vi "ConstantForce.vi"() -> ()   [LabVIEW 2011]
doc: "This example is a template that gives the structure of a single-loop PID controller. This VI uses the PID Filter VI to reduce measurement noise. This VI also uses the PID Autotuning VI to tune the controller based on the closed-loop response. This VI also uses the Timed Loop to ensure deterministic execution.\n\nReplace the Dummy Input and Dummy Output VIs with code that communicates with a real-time target."
uses:
  <vilib>/addons/Digital Filter Design/_Objects.llb/DFD Filter Obj.ctl
  <vilib>/addons/Digital Filter Design/_Objects.llb/DFD Filter Coef.ctl
  <vilib>/addons/Digital Filter Design/_Objects.llb/DFD Filter Structure Type Selector.ctl
  <vilib>/addons/Digital Filter Design/_Objects.llb/dfd_Internal Quantization Settings.ctl
  <vilib>/addons/Digital Filter Design/_Objects.llb/dfd_Internal Quantization Srcs.ctl
  <vilib>/addons/Digital Filter Design/_Objects.llb/DFD Coef Norm Type.ctl
  <vilib>/Platform/TimedLoop/XDataNode/timing_clust.ctl
  <vilib>/Platform/TimedLoop/XDataNode/nitl_modes.ctl
  <vilib>/Platform/TimedLoop/XDataNode/wakeup.ctl
  <vilib>/DAQmx/write.llb/DAQmx Write (Counter Frequency 1Chan 1Samp).vi
  <vilib>/DAQmx/write.llb/DAQmx Write (Digital 1D Bool NChan 1Samp 1Line).vi
  <vilib>/DAQmx/read.llb/DAQmx Read (Counter DBL 1Chan 1Samp).vi
  <vilib>/DAQmx/read.llb/DAQmx Read (Analog 1D DBL NChan 1Samp).vi
  <vilib>/addons/control/pid/pid.llb/PID Advanced (DBL Array).vi
  <vilib>/addons/control/pid/pid.llb/PID Derivative Action Buffered (DBL Array).vi
  <vilib>/addons/control/pid/pid.llb/PID Get Advanced Error (DBL Array).vi
  <vilib>/addons/control/pid/pid.llb/PID Integral Action Buffered (DBL Array).vi
  <vilib>/addons/control/pid/pid.llb/PID Resize 1D Array.vi
  <vilib>/addons/control/pid/pid.llb/PID Get Advanced Error (DBL).vi
  <vilib>/DAQmx/create/channels.llb/DAQmx Create Channel (CO-Pulse Generation-Frequency).vi
  <vilib>/DAQmx/configure/timing.llb/DAQmx Timing (Implicit).vi
  <vilib>/DAQmx/miscellaneous.llb/DAQmx Fill In Error Info.vi
  <vilib>/addons/Digital Filter Design/Process.llb/DFD Filtering (PtByPt NChan).vi
  <vilib>/addons/control/pid/pid.llb/PID Parameter Manager (DBL Array).vi
  <vilib>/measure/maspectr.llb/FFT Spectrum (Mag-Phase) for 1 Chan.vi
  <vilib>/Platform/TimedLoop/XDataNode/XDataNode.xnode
  <vilib>/Platform/TimedLoop/XDataNode/XDNodeRunTimeDep.lvlib
  <vilib>/addons/Digital Filter Design/NI_DigFilterLicensed.lvlib
  <vilib>/measure/NI_MAPro.lvlib
  <vilib>/Analysis/NI_AAL_SigProc.lvlib
  <vilib>/addons/control/pid/NI_PID_pid.lvlib
panel:
  in  "linearity":dbl=1.0 format="%.2f"
  out "PIDGainsOut":T1(array[cluster])=[{"proportional gain (Kc)"=0.30000000000000004, "integral time (Ti, min)"=0.0, "derivative time (Td, min)"=0.0}, {"proportional gain (Kc)"=0.30000000000000004, "integral time (Ti, min)"=0.0, "derivative time (Td, min)"=0.0}, {"proportional gain (Kc)"=0.30000000000000004, "integral time (Ti, min)"=0.0, "derivative time (Td, min)"=0.0}]
  in  "PIDGains":T2={"proportional high (Kc)"=0.5, "integral high (Ti, min)"=0.0, "derivative high (Td, min)"=0.0, "derivative low (Td, min)"=0.0, "integral low (Ti, min)"=0.0, "proportional low (Kc)"=0.1}
  in  "PWMFreq(Hz)":dbl=20000.0 format="%#.6f"
  out "Spectrum":cluster{"f0":dbl, "df":dbl, "magnitude":dbl[]}(graph)={"f0"=0.0, "df"=0.5, "magnitude"=[0.09620328441748356, 0.06810409897269343, 0.0003594915796713484, 0.00021014860402491955, 0.00018846954399764898, 0.000336144679529325, 0.0003012130801723677, 0.00019445462332171186, 0.00033289517846645525, 0.000562837200884615, 0.0006867747058623169, 0.0005811212987675227, 0.00042648431087789106, 0.00036723054948810537, 0.0005888304364960171, 0.0003765129395675796, 0.0002678403496865518, 0.00026380175267942224, 0.000361787601543214, 0.0001537222322813939, 0.0004248104230093206, 0.000271774297036959, 0.00019403766325024087, 7.837182938118593e-05, 0.00024086646260639623, 0.00021325629753186142, 0.00035497074211725515, 0.0005320390408672116, 0.0005154588307424057, 0.000495977514915726, 0.0001925926892680212, 0.00019634614136678798, 0.00046755672378875993, 0.00021183899474091903, 0.000356482164933941, 0.0005724397171551199, 0.0006112453042765386, 0.00014832611393915694, 0.0005354449091516573, 0.0002972453160266781, 0.00017597805789222284, 0.00032530655361426877, 0.00014118024452655864, 0.00036010109356104285, 0.000578316221003946, 0.0007461816021521776, 0.0008385140163832047, 0.0004886726202003539, 0.0003150315464376134, 0.000525543904177902, 0.00041318124423732366, 0.0003192525289590377, 0.00044682022013315406, 0.00023378315775143073, 0.0004028294060579752, 0.00016764084886402385, 0.0002658689552949207, 0.00011811227072949446, 0.0005108675726238193, 0.000528660037898421, 0.0004661368639780102, 0.0001969172989955398, 0.0002997817435090788, 0.0005232481265916394, 0.00029153354829127535, 0.00034458564082988065, 0.0003625549267826836, 0.00030485399320604465, 2.100427401405029e-05, 0.00033163055233150494, 0.0002575243373899191, 0.00031024447712355024, 0.0007095809580562265, 0.0005526875168590069, 0.00018836331735285066, 0.0003619452686631739, 0.0004012983928592705, 0.0003666381061545948, 0.000163582673291403, 0.00012291988292315167, 0.00015891526892010527, 0.00030324875662186086, 0.0001862711270856599, 0.0002485152285499018, 0.0010135478143531338, 0.0008078916475509933, 0.00019359871503329563, 0.000242729443732801, 0.0003349348406560765, 9.595394744410574e-05, 0.00025533462003401097, 0.0001751733067829238, 0.00021051280903753254, 0.0005121321454423101, 0.00027114121521858316, 0.00015587679564032464, 5.8841200038904936e-05, 0.00020608135420260734, 0.00011735729480533824, 0.00010462900746872218, 0.0001985190237984826, 0.00022073477853828147, 0.0003930499011930387, 0.00015089927914282338, 0.00017461102815684548, 0.00036546505890260473, 0.0004575643420051038, 6.526037412657404e-05, 0.00023842870451437197, 0.00022795175255096854, 0.00018803736048158008, 0.00043762334105444596, 0.00037204602762833686, 0.0003858127901442611, 0.00019537399379967473, 0.00030700211982774474, 0.00023405998375632787, 0.0003412354867453395, 0.00030349101678903823, 0.0005609930012192304, 0.0005962425745295062, 0.0022891501106861896, 0.001532704893945848, 0.00038033835660364, 0.0006200757374118415, 0.0004930594092931169, 0.00024339834621575263, 0.0003658239842420277, 0.0005250237628612773, 0.0003061662633654362, 0.0004469940702075021, 0.00045614841528136314, 0.00026832273527844684, 0.0005091044695006741, 0.0003169947020805991, 0.00023486424468684847, 8.763839647824092e-05, 0.00012753416525012625, 0.0003161495448484612, 2.4514922051848186e-05, 0.0002764823360063886, 0.0001578650633790925, 0.00010584168072209294, 0.00014471171973597772, 0.00034066054923323106, 0.00013362866729409327, 0.00033852904863394633, 0.0003590766483400952, 0.00014033182697085645, 0.00011189728703164615, 0.00037718943519435576, 0.0003853277661842273, 0.0001247091613316533, 0.00015688449877991313, 0.0003789219713444136, 0.00018460493488254377, 0.0003119702921186279, 3.0397927282497637e-05, 0.0003359855665221087, 0.0004626969711366938, 0.0003920309415639225, 0.00013392270975849446, 8.86969666433672e-05, 0.00028416480332106846, 0.0004775515986091747, 0.00017753284475210284, 0.00024506374036664647, 0.00046639045447426954, 0.00046301499237699274, 9.541922668358468e-05, 0.0001347948324566838, 2.8572305924906603e-05, 0.00021058685814798146, 0.0003797764082673831, 0.00035629394402777965, 0.00032325251665472844, 0.00040608713555629743, 0.00026898733488955054, 0.0003224959059278195, 0.0004177458017480001, 0.0003681014963565972, 0.00021977425088954856, 0.00035957776746553847, 0.0003226402567141675, 0.00016441447267492444, 0.0002355870386269575, 0.0002162722984969486, 0.0001896749433490035, 4.427063644161406e-05, 0.0002739512902890422, 0.00057854822568849, 0.00033369187305485866, 0.000289470863002901, 8.046137507455306e-05, 0.00023404201343144298, 0.00019294437276071608, 6.054397015157805e-05, 0.00019065185856366197, 0.00027288045779204795, 0.00026849048114022014, 0.00025544691639125465, 0.00013667814777984988, 0.00031897709809037964, 0.0003167770003048542, 0.00018790987805623638, 0.00014065616466841214, 0.00027750941214549823, 0.00034764390165337514, 0.00016498491417466518, 0.00026200335705082545, 0.0002430179402840247, 0.00012993406172108322, 0.00011384517778497205, 0.00020210395661492624, 0.0001926177237363148, 0.0001566807843681054, 8.786807745152152e-05, 0.00011506274315827096, 0.00018052211173992514, 0.0003506426925901174, 0.0001150344595900169, 0.0002006531517296627, 0.00012199567861928173, 6.968881651603949e-05, 0.000146895434695057, 0.00010177868227619922, 7.146367819549118e-05, 0.00012302008869253934, 0.00015391572161203, 0.0003878908024648666, 0.00016205775672610318, 0.0003730406559238256, 0.0004949639629069069, 0.0002414474567828382, 6.715996397035274e-06, 0.0001982056525915547, 0.00017415448516628528, 0.00012697343205469538, 7.0467005193071e-05, 8.522897645077587e-05, 0.00011608238840935515, 0.00021737273984480314, 0.0002143539233942704, 0.0001547982432409731, 0.00013387049192060244, 0.00024362621289604044, 0.00025346685262303667, 0.00011828114208063182, 0.0001410973697475952, 0.00016484708553944803, 9.362003895362505e-05, 3.742238618907275e-05, 8.816624296788719e-05, 8.660419917454452e-05, 8.454844225543479e-05, 0.00014563770331394723, 0.00016165886336021103, 0.00029643091094315444, 0.00022617051620957054, 7.425864446578824e-05, 0.00012984973460739143, 0.00029941459060023215, 0.00019887115018064593, 0.0001550592860894656, 0.00010701912873426859, 5.644325495758224e-05, 0.00012987724039262955, 0.0001623444017767889, 0.0001245355197327217, 0.00014574362683201258, 2.5439415031698453e-05, 8.203135152081712e-05, 0.00011453414541864422, 1.5990912903028797e-05, 9.48759521834382e-05, 8.071394034967105e-05, 0.00017365760224407863, 0.00017999404550366962, 9.887670279700942e-05, 5.502379636777061e-05, 8.329224876693273e-05, 0.00011744377274604075, 0.00012808337474860536, 0.00017429621949908563, 6.559673716533871e-05, 8.517439602839222e-05, 5.581680993555922e-05, 0.0001248433166413104, 0.00011297876140050008, 0.00010607476864400097, 7.557647775344107e-05, 9.027165709926598e-05, 9.26301339988804e-05, 7.111166199659558e-05, 4.503125015873237e-05, 7.134205040841814e-05, 0.00017176642240616653, 0.00015805834772730266, 6.354909821912828e-05, 4.710721765108564e-05, 5.961174275940043e-05, 2.3994340360453395e-05, 2.9612149535282676e-05, 8.068837779654663e-05, 8.337468168258811e-05, 5.9948988957651735e-05, 1.2901070157195641e-05, 9.928627098209403e-05, 9.911589258071182e-05, 9.27104415452593e-05, 5.297783951889115e-05, 8.866164597341511e-05, 6.873540575424902e-05, 2.9752777982596516e-05, 0.00017445943670187227, 0.00024159254243468698, 0.00011658923271226115, 0.00012737326503517066, 0.0001389373667419545, 0.00010623090442469181, 7.523416408699585e-05, 7.220312378677459e-05, 3.864949977027068e-05, 4.515642057022097e-05, 5.204067025147724e-05, 9.064350175867587e-05, 5.107043973201085e-05, 0.0001245826862645853, 0.00010515742874481237, 4.752206290018221e-05, 0.00010955241723395005, 7.407898359610076e-05, 2.1708007746722337e-05, 2.019715590464164e-05, 2.1987406689666923e-05, 5.450113354923983e-05, 7.161957983578496e-05, 6.641173438069711e-05, 6.87976800359608e-05, 5.240743045604911e-05, 3.664493515963725e-05, 7.418481441817933e-05, 9.749743503975909e-05, 9.073727003872781e-05, 2.1989849094629526e-05, 5.746344157877747e-05, 1.8546935661777757e-05, 2.722942258343563e-05, 3.0658397698000485e-05, 9.776292178957533e-06, 1.2335863321959672e-05, 3.2727818473110664e-05, 1.3584172902497782e-05, 1.3556247846696258e-05, 1.2761952374912845e-05, 5.991948995900634e-05, 3.816873057478155e-05, 6.78400724612916e-05, 8.797430347711267e-05, 5.2462210266196544e-05, 1.058840890246386e-05, 2.5716730457104114e-05, 1.2751793024547623e-05, 1.6181032458945755e-05, 2.5965989392743585e-05, 4.399652423913049e-05, 5.88406679814353e-05, 3.9070027684511886e-05, 1.6725512968109914e-05, 1.0581280299026412e-05, 2.744399368794747e-05, 3.794992163132296e-05, 2.366887226580642e-05, 2.7508074750656194e-05, 3.317018088757152e-05, 1.866435406036027e-05, 1.1448271641135718e-05, 1.0825975855801427e-05, 1.9921166088270942e-05, 2.513310121648055e-05, 1.4239372227448338e-05, 1.9887056193184144e-05, 3.146587181328742e-06, 4.3519333042847355e-06, 1.633265643308589e-05, 1.3654781858151129e-05, 3.6984701177022112e-06, 4.393726542097977e-05, 4.816543678632307e-05, 2.734925118918193e-05, 2.1002282860069026e-05, 1.66693272371177e-05, 2.070731099804239e-05, 3.2537835380993076e-05, 2.419553306105436e-05, 4.797854579184654e-06, 2.2696380463346525e-05, 2.783896678820508e-05, 1.370374056458416e-05, 1.2943130388085828e-05, 1.1433275758105753e-05, 1.179814825411713e-05, 1.563252142645715e-05, 1.928199143307197e-05, 1.8918668232749954e-05, 1.1217316209080702e-05, 1.5511054495680417e-05, 6.777718332613398e-06, 1.8789937755635533e-05, 1.7817142540518592e-05, 1.2246089319170154e-05, 1.6629467750457185e-05, 2.051993540859729e-05, 2.098327932203105e-05, 6.057051820967863e-06, 6.714391983681018e-06, 6.356643139768899e-06, 8.45582646188679e-06, 5.622569738697892e-06, 1.101240684909168e-05, 1.4877549032696077e-05, 1.1375986593766988e-05, 2.1919217303393563e-05, 9.085871491365278e-06, 7.113283544734878e-06, 8.90330457997047e-06, 4.204796216997096e-06, 3.146586604005787e-06, 1.1864122475267509e-05, 8.031106867579854e-06, 1.673194894661554e-05, 1.4838719535550372e-05, 7.676926094324783e-06, 9.075501319720288e-06, 1.1944944178936969e-05, 1.474485000341705e-05, 1.2708533924253252e-05, 7.69134264262961e-06, 9.227018347894073e-06, 9.212924339304453e-06, 3.328667065598246e-06, 1.2192521743742533e-06, 6.243367757449738e-06, 8.145248483128033e-06, 4.198918661045435e-06, 3.4536181503597517e-06, 2.876059688420414e-06, 3.905495276080273e-06, 1.4292042475222298e-06, 8.479636863469126e-06, 9.210340389267687e-06, 5.605733075526359e-06, 3.790261615336645e-06, 9.418746953239675e-06, 7.085601974602631e-06, 3.0766303720674894e-06, 3.3052793820751635e-06, 2.8546269877500196e-06, 2.51701206501622e-06, 1.8052139276980944e-06, 1.7403829578077524e-06, 1.0584944017724884e-06, 1.6725816625413308e-06, 3.307333766032992e-07, 2.9967094274224586e-06, 3.877751092725656e-06, 1.8869262207121956e-06, 1.2752257736566088e-06, 1.9642704077222505e-06, 1.0701563578186096e-06, 1.991003772579639e-06, 1.1607729113388639e-06, 1.4981891685177038e-06, 1.7766857493655908e-06, 1.573352882509041e-06, 6.17712818164893e-07, 9.452628796891533e-07, 6.780960114057853e-07, 7.406728534477673e-07, 8.039180288673095e-07, 1.063098315213064e-06, 8.620397016686821e-07, 3.147087969268049e-07, 1.981102915309727e-07, 3.7101935446433206e-07, 6.138210777301254e-08, 1.89995686915322e-07, 4.2804403030564556e-07, 4.1689177227729523e-07, 1.7798343882459082e-07, 7.86936916014098e-08, 1.462621897938822e-07, 1.958000307955489e-07, 1.8085415729356566e-07, 5.1844510886849234e-08, 4.407352580185888e-08, 3.1182796069226113e-08, 2.3418690476252897e-08, 1.0829329464468605e-08, 3.6253838968036444e-09]}
  out "EncMax":dbl[](array[numeric])=[6.498, 6.518000000000001, 6.474]
  in  "BndrsCluster":T3={"InwardLimit(%)"=[0.7, 0.7, 0.7], "OutwardLimit(%)"=[0.3, 0.3, 0.3], "SpringCnst"=[5.0, 5.0, 5.0]}
  out "EncPos":dbl[](array[numeric])=[5.53125, 5.478, 5.5135000000000005]
  out "LP_LoadCell":T4={"mSRate_Fs"=500.0, "mSRate_Version"="2.0", "mSRate_Comments"="", "mSRate_OrgCoef"={"type"=enum."IIR Cascaded Second Order Sections Form II Transposed", "gain"=1.0, "coef a (k)"=[-0.36952737735124136, 0.1958157126558331], "coef b (v)"=[0.20657208382614797, 0.41314416765229595, 0.20657208382614797]}, "mSRate_CurCoef"={"type"=enum."IIR Cascaded Second Order Sections Form II Transposed", "gain"=1.0, "coef a (k)"=[-0.36952737735124136, 0.1958157126558331], "coef b (v)"=[0.20657208382614797, 0.41314416765229595, 0.20657208382614797]}, "mSRate_Quantized?"=FALSE, "mSRate_QCoef"={"type"=enum."Undefined", "gain"=1.0, "coef a (k)"=[], "coef b (v)"=[]}, "mSRate_QSettings"=[], "mSRate_Order"=2, "mSRate_Scaling"={"mSRate_ScaleByPowerOf2?"=FALSE, "mSRate_ScaleType"=enum."No Norm"}} {"mSRate_QSettings"."source" items=["Coef a/k"=0, "Coef b/v"=7, "Input"=1, "Output"=2, "Multiplicand"=3, "Product"=4, "Sum"=5, "Delay"=6, "Gain"=8]}
  in  "LP_LoadCell(Hz)":dbl=100.0
  out "Peaks":cluster{"Locations":dbl[], "Amplitudes":dbl[]}
  out "MotorDir":bool[](array[boolean])=[FALSE, TRUE, TRUE]
  in  "ChartLength":dbl=2000.0
  out "FFTArray":dbl[](array[numeric])=[0.09102094165909652, 0.08880080695999211, 0.08742537267011773, 0.08903439623636634, 0.09196169234838143, 0.09470367128274114, 0.09783665070128943, 0.09789838144314505, 0.09594205914249723, 0.09363339103027582, 0.09111500840178702, 0.09203831504284742, 0.09713069022987347, 0.10134606515787001, 0.10061861907733752, 0.09843897276856389, 0.09804067529312961, 0.09755044051782759, 0.0976403166754025, 0.09725636922533248, 0.09471411781510511, 0.09289638367605484, 0.09463637756896869, 0.10108862118124308, 0.10335985683317359, 0.09643477655571013, 0.09248787564173953, 0.09323062466464398, 0.09304905947987505, 0.09264978533169155, 0.09214417573397773, 0.09390841780702704, 0.09540399956340267, 0.09227373877182224, 0.09095729107756384, 0.09392871530582937, 0.0943702886709022, 0.08818127732286983, 0.0807007270500169, 0.08222546366236534, 0.09239407386402292, 0.10311749567286, 0.10471285762085267, 0.0964395109898104, 0.09034274660193076, 0.08915833478556265, 0.08816672057416365, 0.09132499663965439, 0.09827291267684694, 0.1000111309712641, 0.0980408243845543, 0.09529649141150409, 0.09168769480452336, 0.09175909791948443, 0.09571722605296652, 0.10078396610263962, 0.10337942605788164, 0.1014243160339357, 0.0973879688812122, 0.09262209630248038, 0.09031450404738024, 0.09331444243965803, 0.09853176609365545, 0.09611436535238259, 0.0883462084018524, 0.09316531134912277, 0.10558468641824159, 0.10678886347597229, 0.09760830011954734, 0.09111787329777818, 0.0897474453433214, 0.09177388258440985, 0.09614267796476492, 0.09981294892553577, 0.10684721226661176, 0.1078320930394148, 0.0968659399944411, 0.0925416262100675, 0.10030149307473206, 0.10238166455529184, 0.09521176688144757, 0.09585474281406252, 0.10141419849985543, 0.10250775879644676, 0.10131637786742215, 0.09823895961308332, 0.09987441648394499, 0.10271171935070175, 0.09869498899095455, 0.09802502865960976, 0.1013086559148363, 0.09767917025294583, 0.0903655011057841, 0.08830538594258142, 0.09119640016394422, 0.09324595223234786, 0.0945781693605675, 0.0961364777205373, 0.0973689435310479, 0.0981906075001171, 0.09650428184662667, 0.09320201923696174, 0.09218527453800356, 0.0928641968506453, 0.08880772620180627, 0.08549814225091175, 0.0918160400789082, 0.09924044045331475, 0.1006880024780284, 0.09709457652728365, 0.09175252607866341, 0.08881311705339597, 0.08676962298788296, 0.08909276722465459, 0.09745872636630303, 0.10002363387018202, 0.09474941391798437, 0.09479589463639002, 0.10619301053989326, 0.11013974313018808, 0.09810776285710797, 0.09159224898156491, 0.09454586178729105, 0.09738746387133843, 0.09683758569714396, 0.09317703251887542, 0.09145502676796455, 0.09195341475060125, 0.09183726851232944, 0.09314903943899071, 0.09621764664922357, 0.10006496184605966, 0.1086383293940109, 0.11026483076134179, 0.09740502737526889, 0.08962730114947677, 0.09204878325853857, 0.0965956485415745, 0.09926388339064521, 0.09908199133688707, 0.10311544290730992, 0.10622108107448491, 0.10065490376453218, 0.09399221564191973, 0.09082253310177452, 0.09271102497698457, 0.1012525124499937, 0.10602868530341275, 0.1026722749787491, 0.10319758832877436, 0.1036662954376473, 0.09813164549595414, 0.09820127558939208, 0.09874362737972482, 0.09261795007496774, 0.0925548637284494, 0.09688408303332961, 0.0931475786261286, 0.0874255261985941, 0.08857582919835429, 0.09211457350330834, 0.09393722111205698, 0.09662856411913412, 0.10123111196606292, 0.10296596776556342, 0.09836056791312328, 0.09235906685147227, 0.09028608175232539, 0.09426437771841292, 0.1001298758773979, 0.10379001436697999, 0.10384108815645533, 0.09815350124546153, 0.09463245337646703, 0.09495433061374936, 0.09248312317373729, 0.08821395727649654, 0.09073953337473195, 0.11323141000634579, 0.12885170155313352, 0.11310065142851995, 0.09769712603806086, 0.09064228954662149, 0.08669795029054495, 0.09082560583271858, 0.09294253567100298, 0.09080399783545823, 0.09192238471589097, 0.09646212722798142, 0.09897805347628216, 0.10431964577385561, 0.10970370530272601, 0.10447413729321658, 0.0959824501621602, 0.0937564320831249, 0.09555675083496182, 0.09843334250128712, 0.10010272181170206, 0.09739437719983716, 0.09394850769089175, 0.09312455120007386, 0.09252291619942024, 0.09219859129440382, 0.09330029323013085, 0.09635625418417197, 0.09989377979578923, 0.09707740950360141, 0.0825286400290957, 0.0742116515981123, 0.0835614097568316, 0.08967018271289941, 0.08809761919163403, 0.0899393812674251, 0.09601098267213592, 0.10044097204337782, 0.09885423777819236, 0.09531572484531821, 0.09436358572146161, 0.0950122057032307, 0.09464476199601543, 0.0947150937691509, 0.09536558141734598, 0.09589427668828288, 0.09526844145691217, 0.09206680991571439, 0.09024003039093455, 0.09227319889926314, 0.09694714177637125, 0.10013985115058632, 0.09927970382273595, 0.10003415571128227, 0.10652988935956782, 0.10576392054710738, 0.09458357237591669, 0.09132343408427156, 0.09539181733336558, 0.0983186064913613, 0.10242688312844601, 0.10440435360069594, 0.10006353383872878, 0.09603975944753498, 0.09566845237077003, 0.09445646943948487, 0.0937258427916497, 0.096498399173728, 0.09934752344549783, 0.0990571102573801, 0.09550810506979841, 0.09029380751494616, 0.09042573958060648, 0.09386549349043373, 0.09458778223341384, 0.10046364491796721, 0.10786347691619338, 0.10438883183150918, 0.09842565593409977, 0.09948204841067702, 0.10101784574352315, 0.09750221132446843, 0.09253571579725435, 0.08956807568195971, 0.08996922635990895, 0.09433244803273629, 0.0981400001262236, 0.09730951016555453, 0.09498002406290165, 0.09550454698949373, 0.09548292078434514, 0.09344281054064055, 0.09411914317897263, 0.09732202289260564, 0.09889327555577414, 0.09671120193041986, 0.09441990679723493, 0.09342686394131444, 0.091365411976931, 0.09050845132446485, 0.09534263430143414, 0.10306713778181106, 0.10450584487448797, 0.0990234509740975, 0.09084127256203062, 0.08709369142597481, 0.09021656273727405, 0.09181028260020982, 0.09109823283902471, 0.09044727443610756, 0.09251548654394454, 0.09736503986769181, 0.09901179246490464, 0.09671517642563755, 0.09518087378212874, 0.09586163678264449, 0.09648979737720542, 0.09725576734099747, 0.09719171821726084, 0.09723530353050332, 0.098663678328929, 0.09773982233939164, 0.09515580263043158, 0.09465776080429732, 0.09400629716840968, 0.09022515258196406, 0.08947371447551435, 0.09513694728563658, 0.09811254490785551, 0.09620635414337135, 0.09507651859514187, 0.0945267183869635, 0.09382421725979852, 0.0956459361826017, 0.09791579910376325, 0.09561349463035275, 0.09394343712503771, 0.09541610000519386, 0.09347644946854719, 0.0897683685757062, 0.0882604517220544, 0.08974524575043759, 0.09617177978036573, 0.10785004696265986, 0.11303390708229241, 0.10597687870653058, 0.10151283573345282, 0.1009344792379192, 0.09784368867081476, 0.09904071888600943, 0.10349669840280362, 0.1040942209998349, 0.10148782505936726, 0.09657490042623461, 0.09314115873421659, 0.09476689178493831, 0.09736746158346737, 0.09940753670154678, 0.10763997903819085, 0.11479529854711948, 0.1069768316687588, 0.09678246562153861, 0.09437403607619825, 0.08991926190075022, 0.08464072873932871, 0.0838422049156726, 0.08585411986322508, 0.09270974096714582, 0.09842968109345317, 0.09900983413969505, 0.0977284165379058, 0.09370619379559553, 0.09096138996160992, 0.0927353404991053, 0.09549410171143649, 0.09741545780358865, 0.09850179236874584, 0.09753334029902613, 0.0938944804227653, 0.09095421884359461, 0.09176025760176629, 0.09470966226615142, 0.09819729499972707, 0.10092611404338708, 0.10287110068670076, 0.1027962250137489, 0.0978173622830017, 0.09254050160889164, 0.09136446540164815, 0.09231575018234112, 0.09434223474076338, 0.09602581659968036, 0.09496820926423802, 0.09116816115664508, 0.08735998487494422, 0.08701165052963132, 0.0918752420339039, 0.09535937616272426, 0.09170292684335234, 0.08637152315549343, 0.09056762543199076, 0.10125595578883476, 0.10271469202300029, 0.09775950759891888, 0.09454609145608173, 0.09306695582041324, 0.09377828073481509, 0.09588077835169251, 0.0979142076883873, 0.09882700945913166, 0.09933648933168406, 0.099033187772869, 0.09653834537480366, 0.09303951793244071, 0.09170465830988545, 0.0941457996614852, 0.09809651341412748, 0.09818062942287485, 0.09582697341162467, 0.09876838394989043, 0.10546921279135386, 0.10275346946121104, 0.09194145449807363, 0.0898225988833451, 0.092125626983029, 0.09370523623585021, 0.09919143901749372, 0.1041951636993691, 0.1066806743004945, 0.10416052948131936, 0.09792099668505777, 0.0952797809377209, 0.09566488601699888, 0.09765147292508924, 0.10113211837654253, 0.10299017639955342, 0.10366729558308667, 0.10191018057912563, 0.09649506988129782, 0.09389071214465278, 0.09557003425213123, 0.09675362737028138, 0.09448731542418246, 0.09265805501182751, 0.09330679658333524, 0.09198404724267795, 0.09127001888440069, 0.09226181555741168, 0.09234502799301768, 0.09219260874297533, 0.09453712895651711, 0.10177796737055392, 0.10958340153225894, 0.10975413491769775, 0.10248466010004485, 0.09536732020150841, 0.09120648811873355, 0.09184800643569438, 0.0986821321253647, 0.10626473072965756, 0.10537453718446824, 0.09520288322362136, 0.08904581063864876, 0.09132773436696105, 0.09514741844304171, 0.09749575758565918, 0.09770635670783624, 0.09799993015447016, 0.09951651213649035, 0.0995205342643167, 0.09687835611906422, 0.09357010582888718, 0.0885918098064579, 0.08590153653140457, 0.09300058682888698, 0.10077446286178039, 0.09991133951530635, 0.09560751560574979, 0.091214169602366, 0.08723907760025741, 0.08892627554995633, 0.09644549844999885, 0.10032051369342253, 0.09912534271581792, 0.09915992139838321, 0.09921451306525575, 0.09778223224387768, 0.09717830735035844, 0.09588013614993547, 0.0927780200018827, 0.09185512397969973, 0.09542549643518046, 0.10008272634984831, 0.10116817181133533, 0.09777543290620841, 0.09466137486733109, 0.09592060890150078, 0.09823504847463188, 0.10058777942336122, 0.10237950070466754, 0.10291698250275211, 0.10768901733126822, 0.10885439884737656, 0.09993104128484098, 0.09276540111803068, 0.09186436245127866, 0.09278994548771279, 0.09166516641293293, 0.09228869480917856, 0.0971713653637861, 0.09912513860644213, 0.09791813921378399, 0.09619280883929195, 0.09366600704017955, 0.09261344714559394, 0.09503915956804532, 0.0981984537879128, 0.09992496692007144, 0.10029654314248054, 0.09863461151252964, 0.09767691053553712, 0.10129973257952882, 0.10181786448461859, 0.09380545602539495, 0.09166428615872282, 0.10000876289467604, 0.10461129330592896, 0.10091426652576975, 0.09590902708070043, 0.09107718711458933, 0.08849791000210501, 0.09200138898585147, 0.09615962040336506, 0.09800372498507702, 0.09893065057675744, 0.0983955647047802, 0.09876634377612285, 0.10151929001679223, 0.10142412979690257, 0.09873475610715217, 0.09890105704989277, 0.09902227746104335, 0.09874144041158964, 0.09929080648579931, 0.09700621727454077, 0.09396554312862367, 0.09411993528641702, 0.09805078929441152, 0.10094385557815756, 0.0995766211211698, 0.09716790672549175, 0.0931507383918105, 0.09005818765844088, 0.09047072972860055, 0.09209656254058018, 0.0913595214132443, 0.09083708412716954, 0.09633256393122286, 0.10087922683078064, 0.10007708228545206, 0.0964043140555525, 0.09289043553835055, 0.09278715599047352, 0.09355315634006024, 0.09450708646843198, 0.10020802674913763, 0.10439641118267241, 0.10017050640257566, 0.09696154696372317, 0.09856007457682515, 0.09758362764252046, 0.09301238360933117, 0.09208989460000822, 0.09535103523500486, 0.09704488040248786, 0.09649501624947075, 0.09292136947127232, 0.08762683169458144, 0.08807286018124134, 0.09251512532824335, 0.09352523022465763, 0.09482456898370897, 0.09857201880281713, 0.10002741623318949, 0.0992614963411499, 0.09819623421351308, 0.09500221408641796, 0.09101806214044308, 0.09063953610348258, 0.09294804769796418, 0.09618044842316048, 0.09864344832634965, 0.09731409098146067, 0.09275731640689558, 0.08958824930657339, 0.08921529543689591, 0.09008924014780986, 0.0922843798603982, 0.09366216208769575, 0.09558199939758943, 0.09828305461466146, 0.09595370732739364, 0.09169090724242437, 0.09486275276922365, 0.09918003470009631, 0.09588463863675534, 0.09615114899202093, 0.10736894176307686, 0.11426943369080936, 0.10533053641881585, 0.09160572246627915, 0.08553935463051385, 0.0881349187985328, 0.09242294313221106, 0.09337402639419164, 0.09331159712083947, 0.09479064404311334, 0.09484349059638743, 0.09248513554256084, 0.09116154660902528, 0.09085685038813406, 0.09296507129029936, 0.09815989027368009, 0.10195227362645769, 0.10228117738839224, 0.10085835473943733, 0.09751269602240561, 0.09370967555567532, 0.09308864653624445, 0.09809065792911877, 0.10390797237770644, 0.10428729986453797, 0.10484705321736316, 0.1063439573737108, 0.10359279242064043, 0.09924852703831326, 0.0952494758177389, 0.09358370667783035, 0.09489784057415311, 0.09501487632028198, 0.0949785525307149, 0.09702974980573481, 0.09938770889790986, 0.0998162055714144, 0.09843377911152251, 0.09703349670590405, 0.09737469105942545, 0.10041408832460698, 0.10236929336371704, 0.10038794849578446, 0.09549563254588557, 0.09230552912861477, 0.09428579109294094, 0.09733021192971705, 0.10009575535906687, 0.10063699551446069, 0.09840489572564667, 0.09822220083516732, 0.09670831294753654, 0.09206699400033341, 0.09171882085270323, 0.09472323262887117, 0.09469805184174276, 0.09561204111984363, 0.09882415494294253, 0.10089755073599155, 0.1009746372012849, 0.09800452889416644, 0.09404398605476502, 0.09018878155226688, 0.08785389300929711, 0.0892087878331425, 0.09349918860945793, 0.09875258866777097, 0.09728600636028967, 0.08773113491061649, 0.0856815303077994, 0.09392363414267457, 0.09684633020230474, 0.09423852280049147, 0.09341352749318232, 0.09226654402586368, 0.09227710107356496, 0.09271963202497929, 0.08942468552678305, 0.08808004412932355, 0.09082025208462184, 0.0943662584247623, 0.0986132484395693, 0.10278541971811173, 0.10425562139598878, 0.10338672407937001, 0.10069281462171725, 0.09461155564547581, 0.09043898221032887, 0.09086241811178179, 0.0956465654213487, 0.10047432523652337, 0.09874012995090306, 0.09662845273612478, 0.09742358901085837, 0.0954416126025474, 0.0944343225427322, 0.10061701780076883, 0.10282239184753347, 0.09680988544522648, 0.09594049942946489, 0.09952890382137601, 0.09851203949360546, 0.09321353268952194, 0.08874726896721062, 0.08937458303830566, 0.09502426723593145, 0.09704743909405683, 0.09341309909207127, 0.09320657330533846, 0.09541194900634187, 0.09621262807269083, 0.09597209460726519, 0.0948260222868175, 0.09694872112465212, 0.10544860150868023, 0.10962955571826748, 0.10094655844693746, 0.09411998258104398, 0.09602810074338575, 0.09644720495875421, 0.09428721442198901, 0.09214689947843446, 0.08792921462480895, 0.08716373336696479, 0.09197270134951673, 0.09204920268606104, 0.09073306300519976, 0.0939728839595127, 0.09356066685722333, 0.08812625530222079, 0.08846796813662568, 0.09920222450533496, 0.1058252143911878, 0.10188908820115482, 0.09868257472108143, 0.0974471506866546, 0.09586570959738368, 0.09545399635530576, 0.09528028923958379, 0.09603600268580659, 0.09766986117065025, 0.09961126326024015, 0.102743664979939, 0.1017975484717779, 0.09590417887737472, 0.09436986087302418, 0.0960950471893677, 0.09258002402887018, 0.09004428691053806, 0.09505743810555885, 0.09878514128365433, 0.10297684075522308, 0.10611677505693812, 0.10082620695105142, 0.09620687334027836, 0.09310800002970553, 0.09182827527750033, 0.095727744524222, 0.09705375327189339, 0.09458796542608221, 0.09301369005214323, 0.09210520432889652, 0.08993839931550959, 0.08913016197974472, 0.09255624228469467, 0.09975241664086784, 0.10670570585410949, 0.10549643336652603, 0.09861578062160453, 0.09146706187237587, 0.08594071806729495, 0.08518463683142836, 0.08854217583721581, 0.0956823300983743, 0.10118154007919228, 0.09853336945909529, 0.08922985179977319, 0.08315873460741482, 0.08728364339410201, 0.09516133282168092, 0.09881287906379264, 0.09672407737478446, 0.0921373488185896, 0.09041236841979136, 0.09121915468652697, 0.08966211275954464, 0.09075594338729104, 0.09907330650665794, 0.10137052776123553, 0.09380125383649235, 0.09394083443448777, 0.09991051836702212, 0.098914133127104, 0.09474091321489582, 0.09161425833149173, 0.0903816234241194, 0.09213408364075391, 0.09528216461959353, 0.09974635308501201, 0.10296376102767685, 0.09948494250957257, 0.09245409320787697, 0.0847234037653295, 0.08124359196979607, 0.08732159111454053, 0.09312453042992751, 0.09443572094409348, 0.09614806429690329, 0.09811827039050844, 0.09920582650164311, 0.09697117498814982, 0.0916159658944723, 0.0891856040590495, 0.09258576128000563, 0.09850595311479003, 0.10216466234193508, 0.10159404847792461, 0.09813734713893262, 0.09316946471982161, 0.089898245406245, 0.09143198123581918, 0.09608607140091953, 0.09873473423395897, 0.09694929148980345, 0.09669789085980723, 0.09956690918966572, 0.0977729875277695, 0.0923041238418928, 0.09046565059013356, 0.09216640295809489, 0.0959330768646728, 0.10013029478045048, 0.10036419805653103, 0.09737402883495548, 0.09529221761444011, 0.09474517102973008, 0.09517299304482099, 0.0970756321518759, 0.10255745875419961, 0.10794133323694724, 0.10505236763333477, 0.09758183404582535, 0.09518044092000434, 0.09686979136411433, 0.0963564439416678, 0.09593176854266736, 0.09809161877980843, 0.09924108473106583, 0.09921188778060949, 0.09940086043005295, 0.0975288291375136, 0.09337070989200846, 0.09236658901389715, 0.09472263130255579, 0.0968237224024725, 0.09996618180738043, 0.10162032330970641, 0.09956354926862832, 0.0977647659354574, 0.09604223038393135, 0.09382542241699236, 0.0933435847837743, 0.09628226322753937, 0.10836470695266869, 0.1185360866116867, 0.11067474781394153, 0.09722535798812948, 0.09059164647623978, 0.09037033981826824, 0.0922399309267108, 0.09078403611098936, 0.09105698636290141, 0.10376259966062101, 0.11649500331537674, 0.11130322578340691, 0.10170161330836708, 0.09786740170856437, 0.09448847841011596, 0.09104852113042589, 0.09094283375218719, 0.0954029276712423, 0.09824516819295355, 0.09849509459457706, 0.09973739131151854, 0.09774831102631165, 0.0927456448651611, 0.09108519344935982, 0.0920998105659684, 0.09434189366287797, 0.09780729946312651, 0.10036989043082956, 0.10109565912158552, 0.09515305577167105, 0.08736552269450357, 0.0884112935503377, 0.09177082542402804, 0.0941287855547005, 0.09738682229038303, 0.0986266391229788, 0.09859453485538511, 0.09729757794543303, 0.09535369697287284, 0.09491193402856518, 0.09415469374433652, 0.0919245995116571, 0.09260229053425066, 0.09711763046042896, 0.0994603212303976, 0.09848540559686833, 0.09555158263322422, 0.09193674661406673, 0.0912660558768004, 0.0918165368284526, 0.09254400827702049, 0.09586111175301713, 0.09772643877338094, 0.09347792465932281, 0.08884232697038624, 0.08922279597187947, 0.09187463167003444, 0.09629467739771397, 0.09992495848273909, 0.10084749495175446, 0.10510922114203466, 0.10708163951765005, 0.09956989395888909, 0.09332447144951299, 0.09340500283643924, 0.094880302503652, 0.09691342764719751, 0.09899058573507037, 0.09966082620027929, 0.0994892484004143, 0.09879975449547401, 0.09599706963028815, 0.09287049518749299, 0.09279118855764833, 0.0950213123437698, 0.09827611194296731, 0.10118169536703843, 0.10261122865414517, 0.10100060223624563, 0.09609561402187453, 0.09200743121302843, 0.08862116346806512, 0.08646433734107578, 0.09119532618246128, 0.09856972918486451, 0.10021442995888795, 0.09758803531006871, 0.09612123672642862, 0.09793415833895243, 0.09899538949715286, 0.09717460829930598, 0.09579196490738726, 0.09602730553486771, 0.09707847234544234, 0.09819997921636264, 0.09732600104331778, 0.09402548360669662, 0.09226028625168499, 0.09457498381103961, 0.10150378557624333, 0.11125041854722023, 0.11056373305326211, 0.0927818464378579, 0.08175411479726982, 0.08755354766678927, 0.0919741357023542, 0.0934579739365533, 0.09712071873894144, 0.09883277187119353, 0.09422826831892607, 0.09004330059339985, 0.09343182204109886, 0.09572244868720534, 0.09428955402912023, 0.09381445993796159, 0.09480061321748565, 0.09874815315489778, 0.10184085471542625, 0.0987270724155361, 0.09302194541720415, 0.08966533112846485, 0.08800933926523152, 0.08538174293270813, 0.08310551408863133, 0.0888319373985028, 0.10005332755264837, 0.10285518512108545, 0.09873141222733123, 0.0953230356843207, 0.09364591903170218, 0.09362054859116155, 0.09466451600736198, 0.09642449020644978, 0.09916989069119003, 0.10215644387012379, 0.10226405616775242, 0.09876434432117011, 0.09330880795867115, 0.09103536825394845, 0.09626304699088227, 0.10584964653613375, 0.10913250641565027, 0.10441438464989818, 0.10184381876786906, 0.09934814040303097, 0.09485819401222303, 0.09369531581738759, 0.0971066747794125, 0.11050198317269021, 0.1170005254963874, 0.10569386990870762, 0.09940418548326989, 0.09738145361344645]
  in  "LoopFreq(Hz)":dbl=500.0 caption="Set Loop Period (us)"
  in  "SetPoint":dbl[](array[numeric])=[5.0, 5.0, 5.0] min=-10.0 max=10.0 step=1.0
  out "PWMTaskC":refnum<k21>
  out "PWMTaskB":refnum<k21>
  in  "PIDLimit":dbl=0.5 caption="MaxDutyCycle" min=0.0 max=1.0 step=0.01 format="%.2f"
  out "LoopPeriod(s)":dbl=0.002 caption="Loop Period (s)" format="%#_10g"
  out "PWMTaskA":refnum<k21>
  out "LoopDuration(us)":i64=1027 caption="Actual Loop Period (us)"
  in  "stop":bool
  out "SlowLoop":bool
  out "Graph":T10(graph)={7.024469067405356, "SetPointOut"=0.08674999999999766, "output"=0.09102094165909652, "output"=0.01281282497729658}
  # "Use to set force (limits = -10 to 10 lbs)"
  # "index"
  # "middle"
  # "thumb"
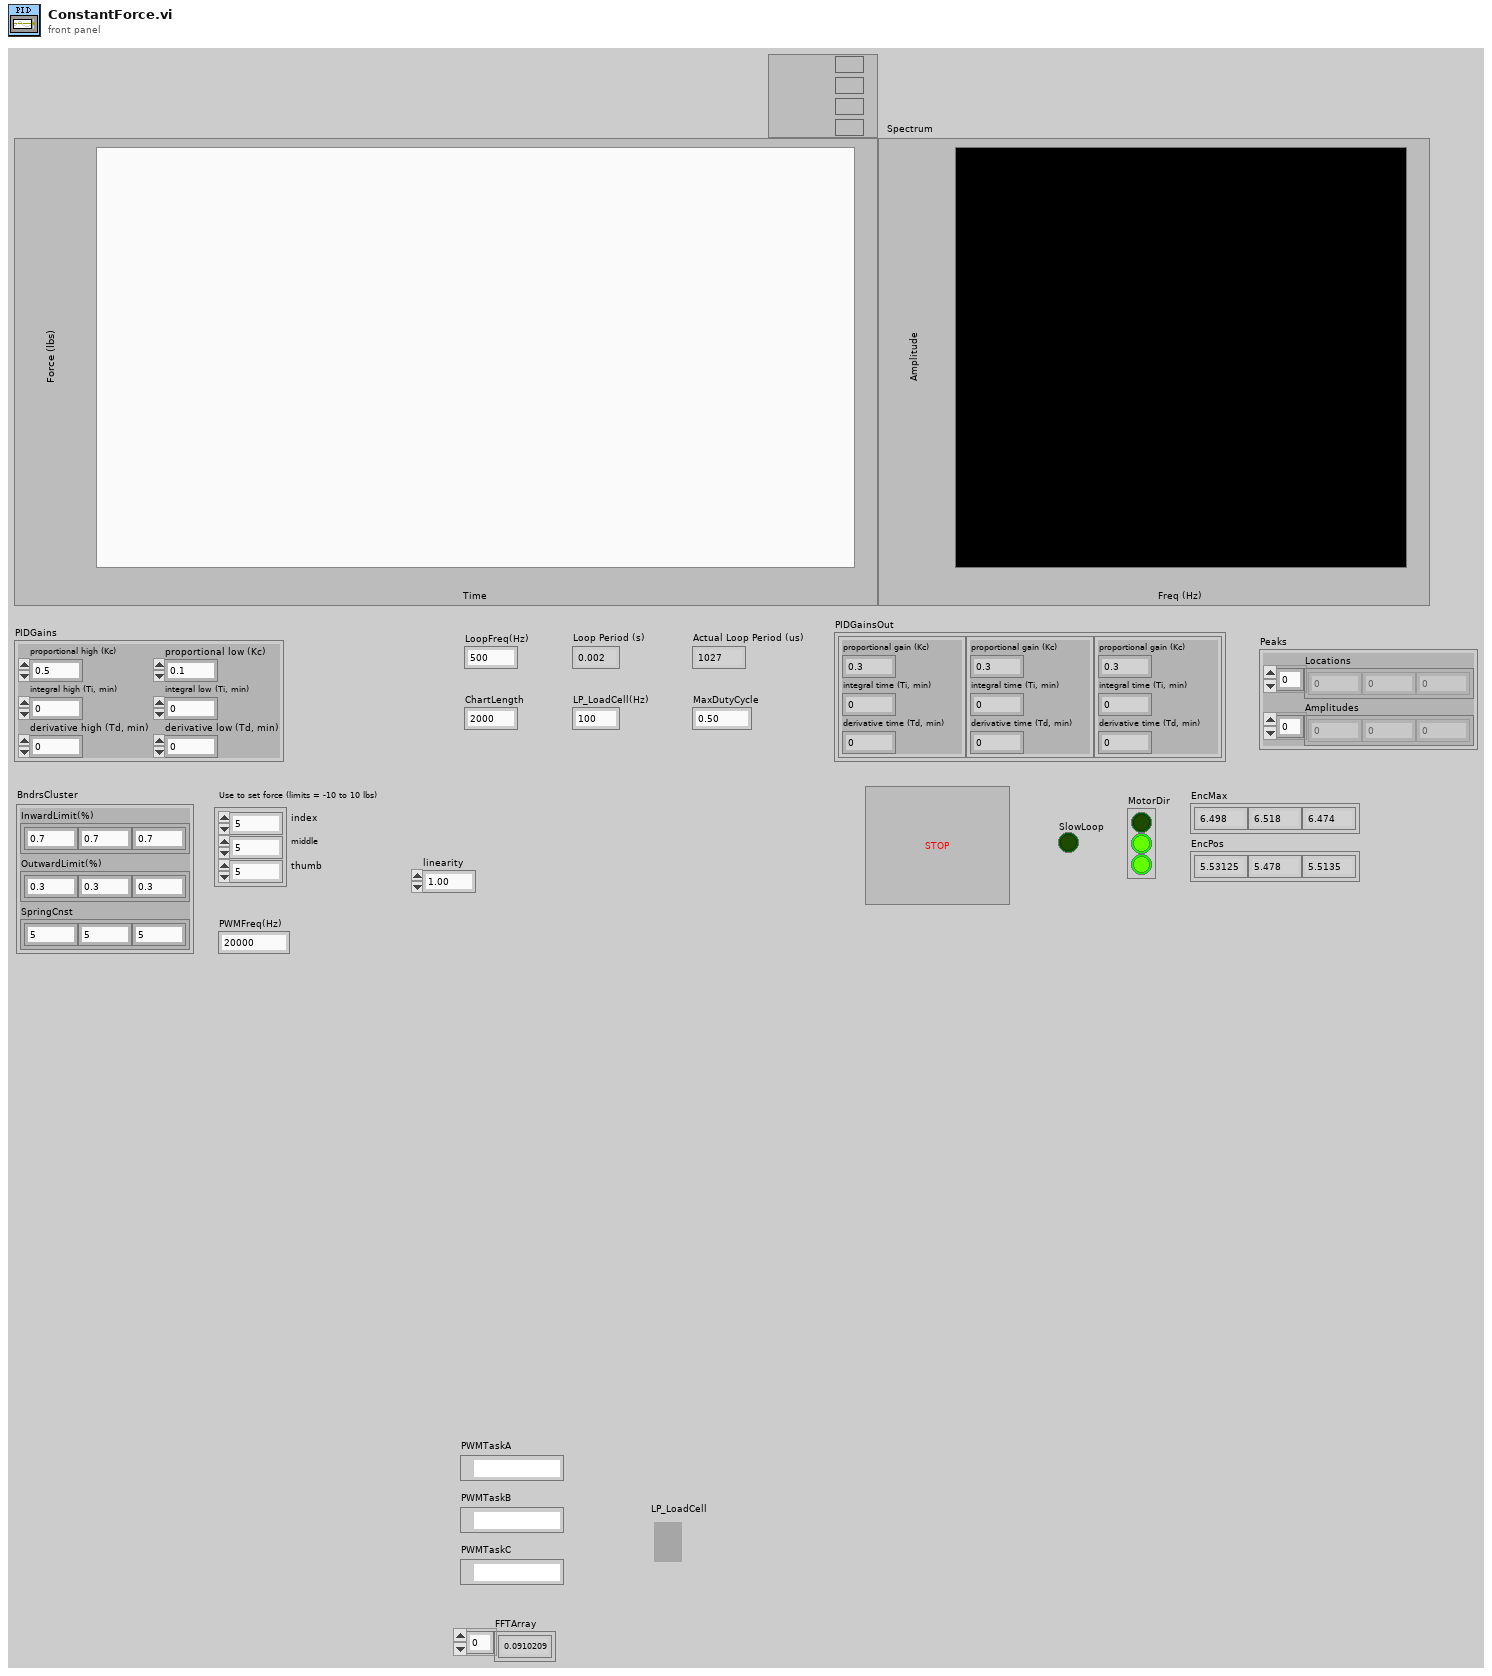
[diagram p1: front panel]
types:
  T1 = cluster{"proportional gain (Kc)":dbl, "integral time (Ti, min)":dbl, "derivative time (Td, min)":dbl}[]
  T2 = cluster{"proportional high (Kc)":dbl, "integral high (Ti, min)":dbl, "derivative high (Td, min)":dbl, "derivative low (Td, min)":dbl, "integral low (Ti, min)":dbl, "proportional low (Kc)":dbl}
  T3 = cluster{"InwardLimit(%)":dbl[], "OutwardLimit(%)":dbl[], "SpringCnst":dbl[]}
  T4 = typedef "NI_DigFilterLicensed.lvlib/DFD Filter Obj.ctl" = cluster{"mSRate_Fs":dbl, "mSRate_Version":string, "mSRate_Comments":string, "mSRate_OrgCoef":T5, "mSRate_CurCoef":T5, "mSRate_Quantized?":bool, "mSRate_QCoef":T5, "mSRate_QSettings":T7[], "mSRate_Order":i32, "mSRate_Scaling":cluster{"mSRate_ScaleByPowerOf2?":bool, "mSRate_ScaleType":T9}}
  T5 = typedef "NI_DigFilterLicensed.lvlib/DFD Filter Coef.ctl" = cluster{"type":T6, "gain":dbl, "coef a (k)":dbl[], "coef b (v)":dbl[]}
  T6 = typedef "NI_DigFilterLicensed.lvlib/DFD Filter Structure Type Selector.ctl" = enum16{"Undefined", "FIR Direct Form", "FIR Direct Form Transposed", "FIR Symmetric", "FIR Antisymmetric", "IIR Direct Form I", "IIR Direct Form I Transposed", "IIR Direct Form II", "IIR Direct Form II Transposed", "IIR Cascaded Second Order Sections Form I", "IIR Cascaded Second Order Sections Form I Transposed", "IIR Cascaded Second Order Sections Form II", "IIR Cascaded Second Order Sections Form II Transposed", "Lattice Allpass (basic sections)", "Lattice Allpass (one multiplier sections)", "Lattice Allpass (normalized sections)", "Lattice AR (basic sections)", "Lattice AR (one multiplier sections)", "Lattice AR (normalized sections)", "Lattice MA (minimum phase)", "Lattice MA (maximum phase)", "Lattice ARMA (basic sections)", "Lattice ARMA (one multiplier sections)", "Lattice ARMA (normalized sections)"}
  T7 = typedef "NI_DigFilterLicensed.lvlib/dfd_Internal Quantization Settings.ctl" = cluster{"source":T8, "wl":i16, "iwl":i16, "overflow mode":enum16{"Saturation", "Wrap"}, "rounding mode":enum16{"Nearest", "Truncation"}, "signed?":bool}
  T8 = typedef "NI_DigFilterLicensed.lvlib/dfd_Internal Quantization Srcs.ctl" = u16
  T9 = typedef "NI_DigFilterLicensed.lvlib/DFD Coef Norm Type.ctl" = enum16{"No Norm", "Time Domain 1-Norm", "Time Domain 2-Norm", "Time Domain Inf-Norm"}
  T10 = cluster{dbl, "SetPointOut":dbl, "output":dbl, "output":dbl}
  T11 = enum16{"Lowpass", "Highpass", "Bandpass", "Bandstop"}
  T12 = typedef "XDNodeRunTimeDep.lvlib/timing_clust.ctl" = cluster{"Expected End [f-1]":u64, "Actual End [f-1]":u64, "Finished Late? [f-1]":bool, "Expected End [i-1]":u64, "Actual End [i-1]":u64, "Finished Late? [i-1]":bool, "Expected Start [i]":u64, "Actual Start [i]":u64, "Expected Start [f]":u64, "Actual Start [f]":u64, "Source Name":string, "Structure Name":string, "Period":i64, "Deadline":i64, "Offset":i64, "Start":i64, "Priority":i32, "Timeout":i32, "Mode":T13, "Wakeup Reason":T14, "Error":errorcluster, "Source Type":string, "Secondary Source Type":string, "Global End Time":u64, "Global Start Time":u64, "Frame Duration":u64, "Iteration Duration":u64, "Assigned CPU":i32, "I/O Scan Engine Mode":u32}
  T13 = typedef "XDNodeRunTimeDep.lvlib/nitl_modes.ctl" = enum32{"No Change", "Process missed periods, maintain original phase", "Discard missed periods, maintain original phase", "Process missed periods, ignore original phase", "Discard missed periods, ignore original phase"}
  T14 = typedef "XDNodeRunTimeDep.lvlib/wakeup.ctl" = enum32{"Normal", "Aborted", "Asynchronous wakeup", "Timing source error", "Timed loop error", "Timeout"}
  T15 = cluster{"element":dbl, "element":dbl, "element":dbl, "element":dbl}
  T16 = cluster{"element":dbl, "element":dbl, "element":dbl, "element":dbl}[]
  T17 = cluster{dbl, "SetPointIn":dbl, "Numeric":dbl, dbl}
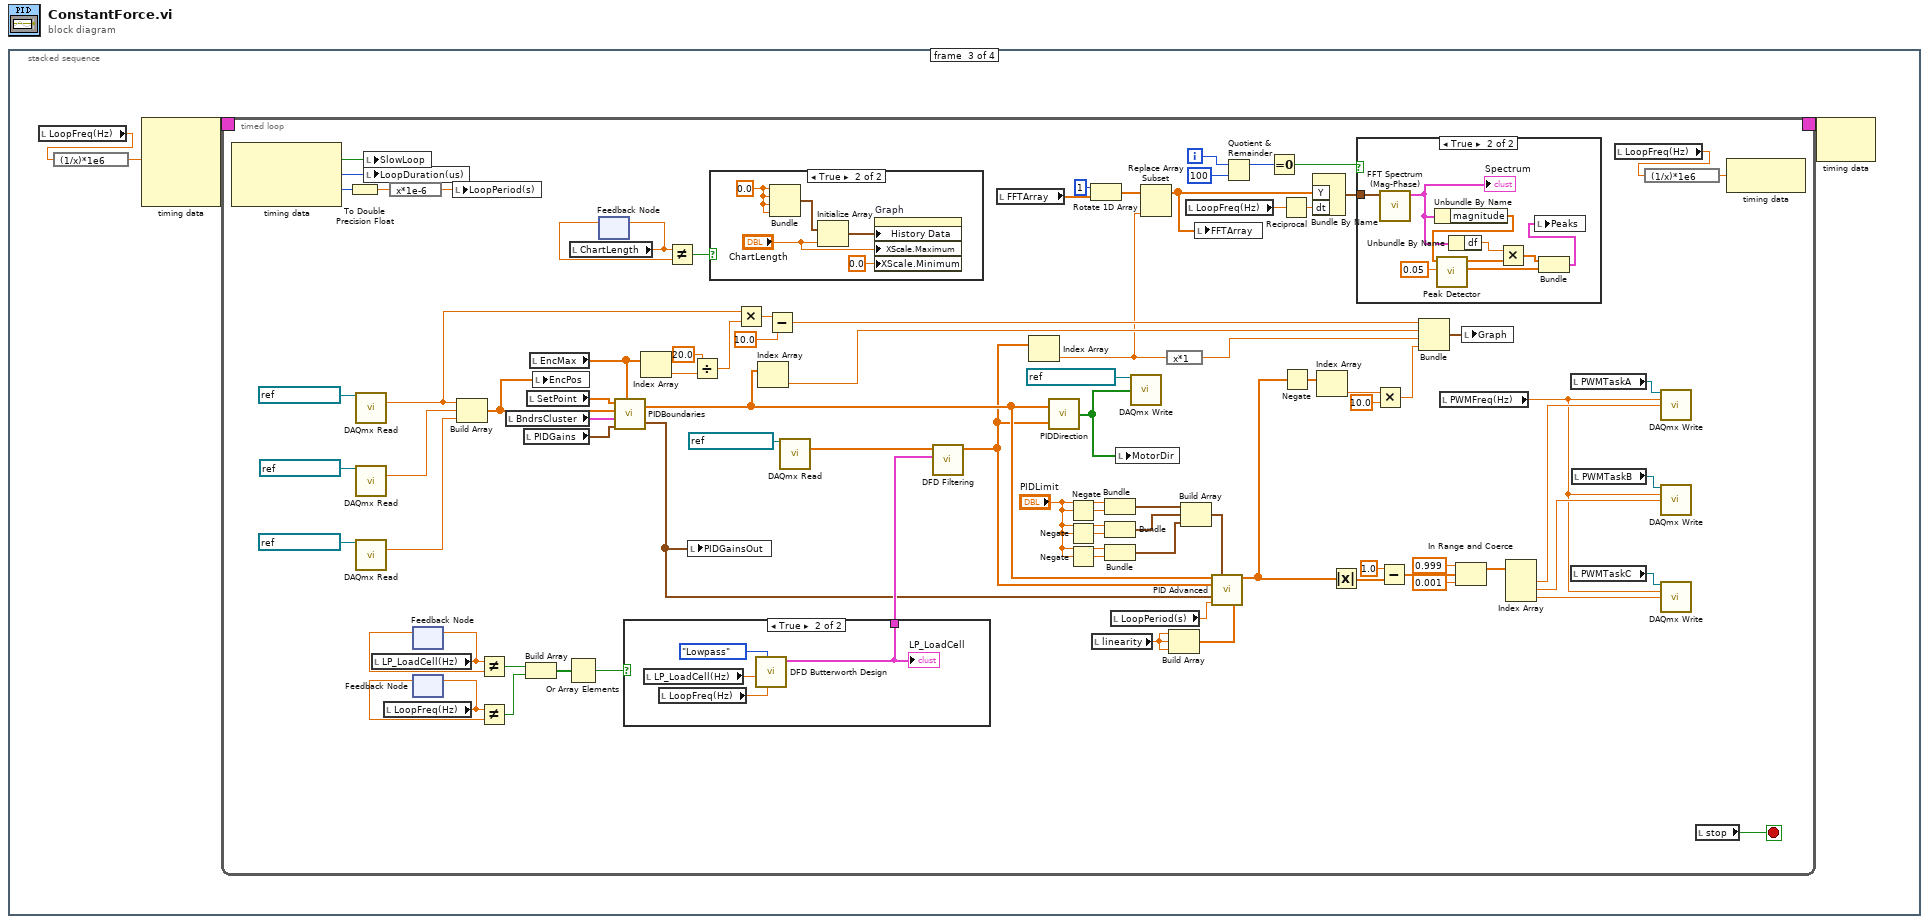
[diagram p0: block diagram]
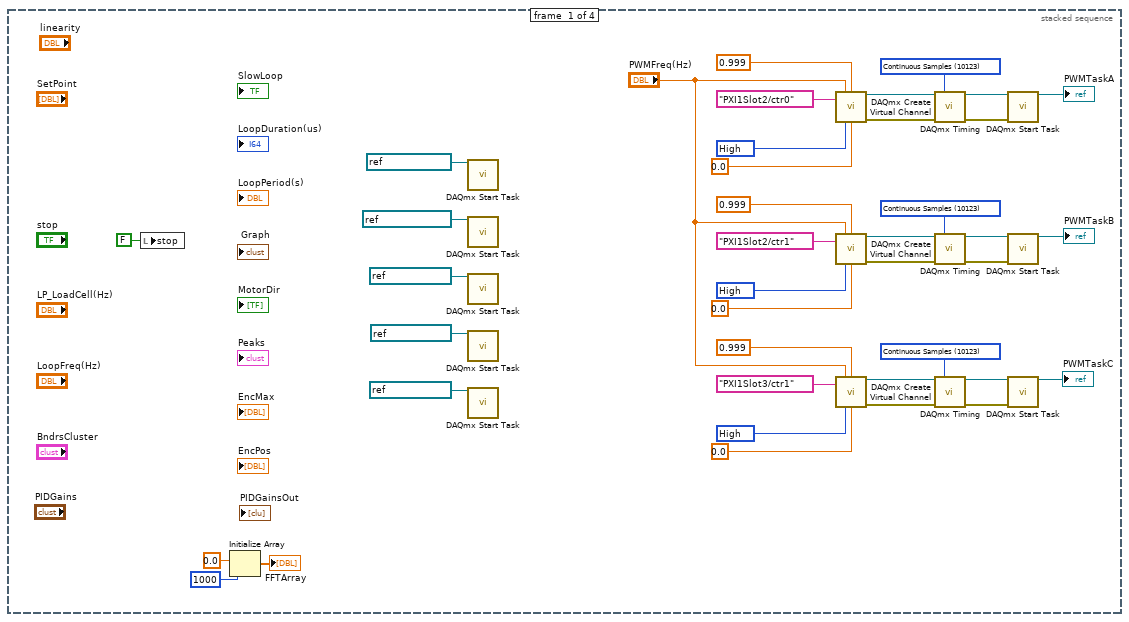
[diagram p2: hidden frame]
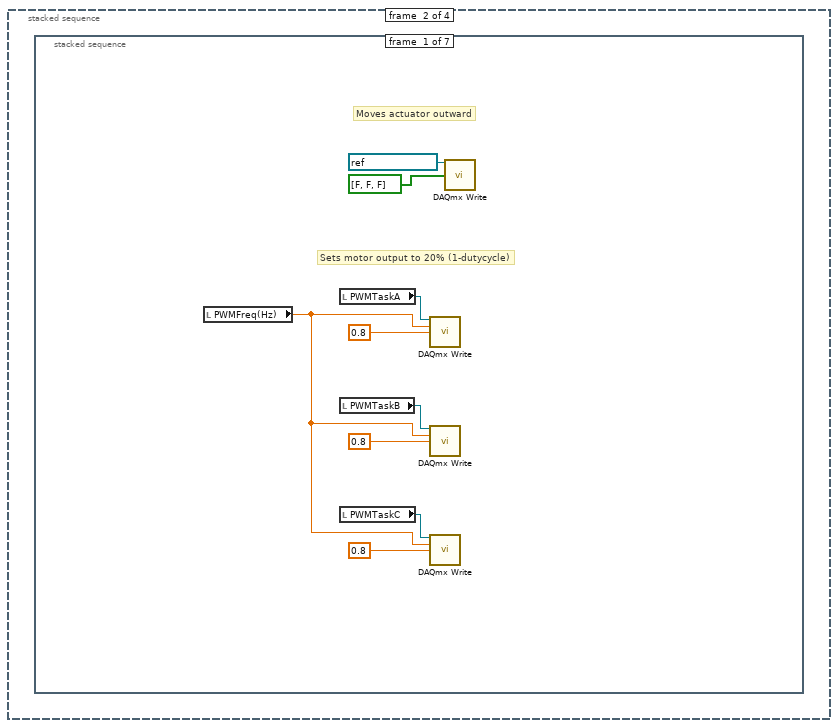
[diagram p3: hidden frame]
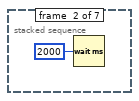
[diagram p4: hidden frame]
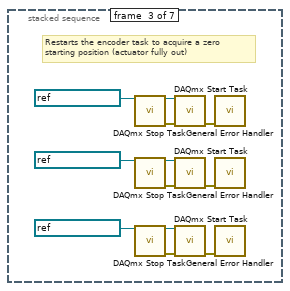
[diagram p5: hidden frame]
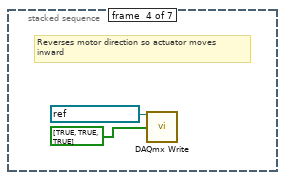
[diagram p6: hidden frame]
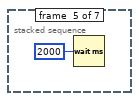
[diagram p7: hidden frame]
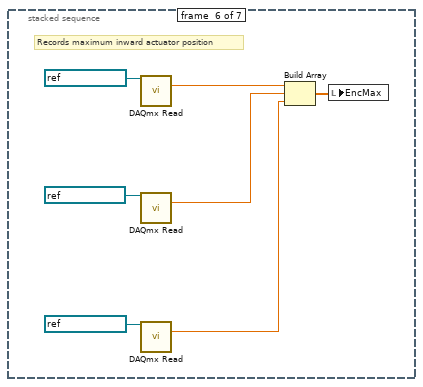
[diagram p8: hidden frame]
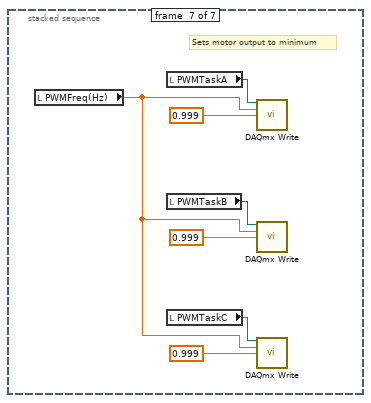
[diagram p9: hidden frame]
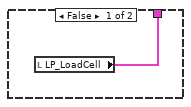
[diagram p12: hidden frame]
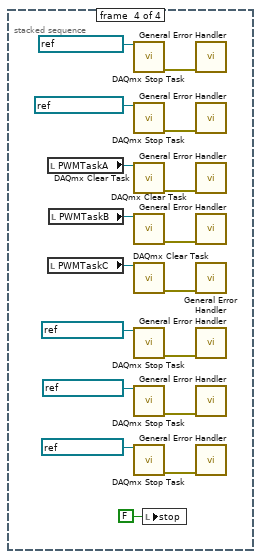
[diagram p13: hidden frame]
diagram:
  n1 = stacked-sequence {
    frame #0 {
      w10 = 10192 items=["High"=10192, "Low"=10214] ("idle state")
      w4 = 10123 items=["Finite Samples"=10178, "Continuous Samples"=10123] ("sample mode")
      w20 = 10192 items=["High"=10192, "Low"=10214] ("idle state")
      w26 = 10123 items=["Finite Samples"=10178, "Continuous Samples"=10123] ("sample mode")
      w37 = 10192 items=["High"=10192, "Low"=10214] ("idle state")
      w30 = 10123 items=["Finite Samples"=10178, "Continuous Samples"=10123] ("sample mode")
      n2 = local write "stop"(FALSE ("stop")) -> ()
      n3 = Initialize Array(0.0, 1000 ("dimension size")) -> (→"FFTArray":dbl[])
      n4 = call <vilib>:"DAQmx Start Task.vi"("task/channels in"=refnum<k21> "ForceInABC") -> ()  [unwired: 13 in, 2 out]
      n5 = call <vilib>:"DAQmx Start Task.vi"("task/channels in"=refnum<k21> "MotorDirABC") -> ()  [unwired: 13 in, 2 out]
      n6 = call <vilib>:"DAQmx Start Task.vi"("task/channels in"=refnum<k21> "PositionInA") -> ()  [unwired: 13 in, 2 out]
      n7 = call <vilib>:"DAQmx Start Task.vi"("task/channels in"=refnum<k21> "PositionInB" ("task")) -> ()  [unwired: 13 in, 2 out]
      n8 = call <vilib>:"DAQmx Start Task.vi"("task/channels in"=refnum<k21> "PositionInC") -> ()  [unwired: 13 in, 2 out]
      n9 = call-poly <vilib>:"DAQmx Create Virtual Channel.vi"("frequency"="PWMFreq(Hz)", "duty cycle"=0.999, "counter"=tag "PXI1Slot2/ctr0", "idle state"=w37, "initial delay"=0.0) -> ("task out"=w33:refnum<k21>, "error out"=w34:errorcluster)  [unwired: 9 in]
      n10 = call-poly <vilib>:"DAQmx Create Virtual Channel.vi"("frequency"="PWMFreq(Hz)", "duty cycle"=0.999, "counter"=tag "PXI1Slot2/ctr1", "idle state"=w20, "initial delay"=0.0) -> ("task out"=w23:refnum<k21>, "error out"=w22:errorcluster)  [unwired: 9 in]
      n11 = call-poly <vilib>:"DAQmx Create Virtual Channel.vi"("frequency"="PWMFreq(Hz)", "duty cycle"=0.999, "counter"=tag "PXI1Slot3/ctr1", "idle state"=w10, "initial delay"=0.0) -> ("task out"=w7:refnum<k21>, "error out"=w8:errorcluster)  [unwired: 9 in]
      n12 = call-poly <vilib>:"DAQmx Timing.vi"("task/channels in"=w33, "sample mode"=w30, "error in"=w34) -> ("task out"=w31:refnum<k21>, "error out"=w32:errorcluster)  [unwired: 11 in]
      n13 = call-poly <vilib>:"DAQmx Timing.vi"("task/channels in"=w23, "sample mode"=w26, "error in"=w22) -> ("task out"=w25:refnum<k21>, "error out"=w24:errorcluster)  [unwired: 11 in]
      n14 = call-poly <vilib>:"DAQmx Timing.vi"("task/channels in"=w7, "sample mode"=w4, "error in"=w8) -> ("task out"=w5:refnum<k21>, "error out"=w6:errorcluster)  [unwired: 11 in]
      n15 = call <vilib>:"DAQmx Start Task.vi"("task/channels in"=w31, "error in"=w32) -> ("task out"=→"PWMTaskA":refnum<k21>)  [unwired: 12 in, 1 out]
      n16 = call <vilib>:"DAQmx Start Task.vi"("task/channels in"=w25, "error in"=w24) -> ("task out"=→"PWMTaskB":refnum<k21>)  [unwired: 12 in, 1 out]
      n17 = call <vilib>:"DAQmx Start Task.vi"("task/channels in"=w5, "error in"=w6) -> ("task out"=→"PWMTaskC":refnum<k21>)  [unwired: 12 in, 1 out]
    }
    frame #1 {
      n18 = stacked-sequence {
        frame #0 {
          # "Sets motor output to 20% (1-dutycycle)"
          # "Moves actuator outward"
          n19 = local read "PWMFreq(Hz)"() -> (w41:dbl)
          n20 = local read "PWMTaskA"() -> (w48:refnum<k21>)
          n21 = local read "PWMTaskB"() -> (w45:refnum<k21>)
          n22 = local read "PWMTaskC"() -> (w42:refnum<k21>)
          n23 = call-poly <vilib>:"DAQmx Write.vi"("task/channels in"=w48, "frequency"=w41, "duty cycle"=0.8) -> ()  [unwired: 10 in, 3 out]
          n24 = call-poly <vilib>:"DAQmx Write.vi"("task/channels in"=w45, "frequency"=w41, "duty cycle"=0.8) -> ()  [unwired: 10 in, 3 out]
          n25 = call-poly <vilib>:"DAQmx Write.vi"("task/channels in"=w42, "frequency"=w41, "duty cycle"=0.8) -> ()  [unwired: 10 in, 3 out]
          n26 = call-poly <vilib>:"DAQmx Write.vi"("task/channels in"=refnum<k21> "MotorDirABC", "data"=bool[] [FALSE, FALSE, FALSE]) -> ()  [unwired: 11 in, 3 out]
        }
        frame #1 {
          n27 = Wait (ms)(milliseconds to wait=u32 2000) -> ()  [unwired: 1 out]
        }
        frame #2 {
          # "Restarts the encoder task to acquire a zero\nstarting position (actuator fully out)"
          n28 = call <vilib>:"DAQmx Stop Task.vi"("task/channels in"=refnum<k21> "PositionInA") -> ("task out"=w60:refnum<k21>, "error out"=w59:errorcluster)  [unwired: 13 in]
          n29 = call <vilib>:"DAQmx Stop Task.vi"("task/channels in"=refnum<k21> "PositionInB") -> ("task out"=w57:refnum<k21>, "error out"=w58:errorcluster)  [unwired: 13 in]
          n30 = call <vilib>:"DAQmx Stop Task.vi"("task/channels in"=refnum<k21> "PositionInC") -> ("task out"=w52:refnum<k21>, "error out"=w51:errorcluster)  [unwired: 13 in]
          n31 = call <vilib>:"DAQmx Start Task.vi"("task/channels in"=w60, "error in"=w59) -> ("error out"=w62:errorcluster)  [unwired: 12 in, 1 out]
          n32 = call <vilib>:"DAQmx Start Task.vi"("task/channels in"=w57, "error in"=w58) -> ("error out"=w55:errorcluster)  [unwired: 12 in, 1 out]
          n33 = call <vilib>:"DAQmx Start Task.vi"("task/channels in"=w52, "error in"=w51) -> ("error out"=w54:errorcluster)  [unwired: 12 in, 1 out]
          n34 = call <vilib>:"General Error Handler.vi"("error in (no error)"=w62) -> ()  [unwired: 10 in, 5 out]
          n35 = call <vilib>:"General Error Handler.vi"("error in (no error)"=w55) -> ()  [unwired: 10 in, 5 out]
          n36 = call <vilib>:"General Error Handler.vi"("error in (no error)"=w54) -> ()  [unwired: 10 in, 5 out]
        }
        frame #3 {
          # "Reverses motor direction so actuator moves\ninward"
          n37 = call-poly <vilib>:"DAQmx Write.vi"("task/channels in"=refnum<k21> "MotorDirABC", "data"=bool[] [TRUE, TRUE, TRUE]) -> ()  [unwired: 11 in, 3 out]
        }
        frame #4 {
          n38 = Wait (ms)(milliseconds to wait=u32 2000) -> ()  [unwired: 1 out]
        }
        frame #5 {
          # "Records maximum inward actuator position"
          n39 = call-poly <vilib>:"DAQmx Read.vi"("task/channels in"=refnum<k21> "PositionInA") -> ("data"=w69:dbl)  [unwired: 12 in, 2 out]
          n40 = call-poly <vilib>:"DAQmx Read.vi"("task/channels in"=refnum<k21> "PositionInB") -> ("data"=w68:dbl)  [unwired: 12 in, 2 out]
          n41 = call-poly <vilib>:"DAQmx Read.vi"("task/channels in"=refnum<k21> "PositionInC") -> ("data"=w67:dbl)  [unwired: 12 in, 2 out]
          n42 = Build Array(w69, w68, w67) -> (w66:dbl[])
          n43 = local write "EncMax"(w66) -> ()
        }
        frame #6 {
          # "Sets motor output to minimum"
          n44 = local read "PWMFreq(Hz)"() -> (w73:dbl)
          n45 = local read "PWMTaskA"() -> (w78:refnum<k21>)
          n46 = local read "PWMTaskB"() -> (w77:refnum<k21>)
          n47 = local read "PWMTaskC"() -> (w74:refnum<k21>)
          n48 = call-poly <vilib>:"DAQmx Write.vi"("task/channels in"=w78, "frequency"=w73, "duty cycle"=0.999) -> ()  [unwired: 10 in, 3 out]
          n49 = call-poly <vilib>:"DAQmx Write.vi"("task/channels in"=w77, "frequency"=w73, "duty cycle"=0.999) -> ()  [unwired: 10 in, 3 out]
          n50 = call-poly <vilib>:"DAQmx Write.vi"("task/channels in"=w74, "frequency"=w73, "duty cycle"=0.999) -> ()  [unwired: 10 in, 3 out]
        }
      }
    }
    frame #2 {
      n51 = local read "LoopFreq(Hz)"() -> (w81:dbl)
      n52 = expression code="(1/x)*1e6"(w81) -> (w80:dbl)
      n53 = node-c288(w80) -> (w83:T12)  [unwired: 3 in]
      n54 = timed-loop {
        timing: w83 -> [_]
        timing-out: [_] -> w82
        i -> [w142]
        stop <- w148 stop-if-true
        n55 = node-c288() -> (w150:bool, w149:i64, w122:i64)  [unwired: 1 in]
        n56 = To Double Precision Float(number=w122) -> (double precision float=w121:dbl)
        n57 = call-poly <vilib>:"DAQmx Read.vi"("task/channels in"=refnum<k21> "PositionInA") -> ("data"=w90:dbl)  [unwired: 12 in, 2 out]
        n58 = call-poly <vilib>:"DAQmx Read.vi"("task/channels in"=refnum<k21> "PositionInB") -> ("data"=w127:dbl)  [unwired: 12 in, 2 out]
        n59 = call-poly <vilib>:"DAQmx Read.vi"("task/channels in"=refnum<k21> "PositionInC") -> ("data"=w126:dbl)  [unwired: 12 in, 2 out]
        n60 = local write "SlowLoop"(w150) -> ()
        n61 = local write "LoopDuration(us)"(w149) -> ()
        n62 = local read "LP_LoadCell(Hz)"() -> (w144:dbl)
        n63 = local read "LoopFreq(Hz)"() -> (w133:dbl)
        n64 = expression code="x*1e-6"(w121) -> (w135:dbl)
        n65 = feedback #1() -> (w143:dbl)  [unwired: 1 in]
        n66 = feedback-in #1(w144) -> ()
        n67 = feedback #2() -> (w134:dbl)  [unwired: 1 in]
        n68 = feedback-in #2(w133) -> ()
        n69 = local write "LoopPeriod(s)"(w135) -> ()
        n70 = Build Array(w90, w127, w126) -> (w123:dbl[])
        n71 = Not Equal?(x=w144, y=w143) -> (x != y?=w132:bool)
        n72 = Not Equal?(x=w133, y=w134) -> (x != y?=w131:bool)
        n73 = local read "BndrsCluster"() -> (w119:T3)
        n74 = local read "PIDGains"() -> (w112:T2)
        n75 = Build Array(w132, w131) -> (w130:bool[])
        n76 = local read "SetPoint"() -> (w120:dbl[])
        n77 = local read "EncMax"() -> (w94:dbl[])
        n78 = local write "EncPos"(w123) -> ()
        n79 = Or Array Elements(Boolean array=w130) -> (logical OR=w129:bool)
        n80 = local read "ChartLength"() -> (w140:dbl)
        n81 = feedback #3() -> (w139:dbl)  [unwired: 1 in]
        n82 = feedback-in #3(w140) -> ()
        n83 = call "PIDBoundaries.vi"("SetPointIn"=w120, "EncPosIn"=w123, "BndrsCluster"=w119, "PIDGainsIn"=w112, "EncMax"=w94) -> ("SetPointOut"=w125:dbl[], "PIDGainsOut"=w111:T1)
        n84 = case shown="True" w129 {
          tunnel: [w186 w187] -> w128
          frame False {
            n85 = local read "LP_LoadCell"() -> (w186:T4)
          }
          frame True {
            n86 = local read "LP_LoadCell(Hz)"() -> (w188:dbl)
            n87 = local read "LoopFreq(Hz)"() -> (w189:dbl)
            n88 = call <vilib>:"DFD Butterworth Design.vi"("fs [Hz]"=w189, "filter type"=T11."Lowpass", "low cutoff freq [Hz]"=w188) -> ("filter out"=w187:T4)  [unwired: 7 in, 1 out]
            "LP_LoadCell" <- w187
          }
        }
        n89 = Index Array(array=w94) -> (element=w93:dbl)  [unwired: 1 in]
        n90 = Not Equal?(x=w140, y=w139) -> (x != y?=w141:bool)
        n91 = local write "PIDGainsOut"(w111) -> ()
        n92 = Divide(x=20.0, y=w93) -> (x/y=w91:dbl)
        n93 = case shown="True" w141 {
          frame False {
          }
          frame True {
            w181 = 0.0 ("element")
            n94 = Bundle("element"=w181, "element"=w181, "element"=w181, "element"=w181) -> (w185:T15)  [unwired: 1 in]
            n95 = Initialize Array(w185, "ChartLength") -> (w182:T16)
            n96 = property on="Graph" class="WFChart (strict)"("History Data"=w182, "XScale.Maximum"="ChartLength", "XScale.Minimum"=0.0 ("X Scale.Range:Minimum")) -> ()  [unwired: 2 in, 2 out]
          }
        }
        n97 = Multiply(x=w90, y=w91) -> (x*y=w89:dbl)
        n98 = Index Array(array=w125) -> (element=w124:dbl)  [unwired: 1 in]
        n99 = Subtract(x=w89, y=10.0) -> (x-y=w87:dbl)
        n100 = call-poly <vilib>:"DAQmx Read.vi"("task/channels in"=refnum<k21> "ForceInABC") -> ("data"=w100:dbl[])  [unwired: 12 in, 2 out]
        n101 = call-poly <vilib>:"DFD Filtering.vi"("filter"=w128, "signal in"=w100) -> ("signal out"=w84:dbl[])  [unwired: 2 in, 7 out]
        n102 = local read "FFTArray"() -> (w104:dbl[])
        n103 = Index Array(array=w84) -> (element=w86:dbl)  [unwired: 1 in]
        n104 = call "PIDDirection.vi"("LoadCellIn"=w84, "SetPointIn"=w125) -> ("MotorDirOut"=w136:bool[])
        n105 = Negate(x="PIDLimit") -> (-x=w163:dbl)
        n106 = Negate(x="PIDLimit") -> (-x=w160:dbl)
        n107 = Negate(x="PIDLimit") -> (-x=w159:dbl)
        n108 = Rotate 1D Array(1:w104, 2:1 ("n")) -> (0:w106:dbl[])
        n109 = local read "linearity"() -> (w99:dbl)
        n110 = Bundle("PIDLimit"="PIDLimit", w163) -> (w158:cluster{"PIDLimit":dbl, dbl})  [unwired: 1 in]
        n111 = Bundle("PIDLimit"="PIDLimit", w160) -> (w157:cluster{"PIDLimit":dbl, dbl})  [unwired: 1 in]
        n112 = Bundle("PIDLimit"="PIDLimit", w159) -> (w156:cluster{"PIDLimit":dbl, dbl})  [unwired: 1 in]
        n113 = local read "LoopPeriod(s)"() -> (w146:dbl)
        n114 = local write "MotorDir"(w136) -> ()
        n115 = call-poly <vilib>:"DAQmx Write.vi"("task/channels in"=refnum<k21> "MotorDirABC", "data"=w136) -> ()  [unwired: 11 in, 3 out]
        n116 = Replace Array Subset(array=w106, new element=w86) -> (w101:dbl[])  [unwired: 1 in]
        n117 = expression code="x*1"(w86) -> (w85:dbl)
        n118 = Build Array(w99, w99, w99) -> (w98:dbl[])
        n119 = Build Array(w158, w157, w156) -> (w147:cluster{"PIDLimit":dbl, dbl}[])
        n120 = local read "LoopFreq(Hz)"() -> (w110:dbl)
        n121 = local write "FFTArray"(w101) -> ()
        n122 = call-poly <vilib>:"PID Advanced.vi"("setpoint"=w125, "output range"=w147, "process variable"=w84, "PID gains"=w111, "dt (s)"=w146, "linearity"=w98) -> ("output"=w116:dbl[])  [unwired: 8 in, 1 out]
        n123 = Quotient & Remainder(x=w142, y=100) -> (x-y*floor(x/y)=w108:i32)  [unwired: 1 out]
        n124 = Equal To 0?(x=w108) -> (x = 0?=w109:bool)
        n125 = Reciprocal(x=w110) -> (1/x=w103:dbl)
        n126 = Negate(x=w116) -> (-x=w114:dbl[])
        n127 = Bundle By Name("Y"=w101, "dt"=w103) -> (w102:waveform(dbl))  [unwired: 1 in]
        n128 = Index Array(array=w114) -> (element=w97:dbl)  [unwired: 1 in]
        n129 = Absolute Value(x=w116) -> (abs(x)=w145:dbl[])
        n130 = case shown="True" w109 {
          tunnel: w102 -> [_ w180]
          frame False {
          }
          frame True {
            n131 = call-poly <vilib>:"FFT Spectrum (Mag-Phase).vi"("time signal"=w180) -> ("magnitude"=w173:cluster{"f0":dbl, "df":dbl, "magnitude":dbl[]})  [unwired: 6 in, 4 out]
            "Spectrum" <- w173
            n132 = Unbundle By Name(w173) -> ("magnitude"=w179:dbl[])
            n133 = call <vilib>:"Peak Detector.vi"("threshold"=0.05, "X"=w179) -> ("Amplitudes"=w177:dbl[], "Locations"=w176:dbl[])  [unwired: 5 in, 3 out]
            n134 = Unbundle By Name(w173) -> ("df"=w172:dbl)
            n135 = Multiply(x=w172, y=w176) -> (x*y=w175:dbl[])
            n136 = Bundle(w175, "Amplitudes"=w177) -> (w174:cluster{dbl[], "Amplitudes":dbl[]})  [unwired: 1 in]
            n137 = local write "Peaks"(w174) -> ()
          }
        }
        n138 = Multiply(x=w97, y=10.0) -> (x*y=w96:dbl)
        n139 = Subtract(x=1.0 ("y"), y=w145) -> (x-y=w169:dbl[])
        n140 = Bundle(w87, "SetPointIn"=w124, "Numeric"=w85, w96) -> (w113:T17)  [unwired: 1 in]
        n141 = local read "PWMFreq(Hz)"() -> (w115:dbl)
        n142 = In Range and Coerce(upper limit=0.999, x=w169, lower limit=0.001) -> (coerced(x)=w154:dbl[])  [unwired: 1 out]
        n143 = local write "Graph"(w113) -> ()
        n144 = Index Array(array=w154) -> (element #1=w153:dbl, element #2=w152:dbl, element #3=w151:dbl)  [unwired: 3 in]
        n145 = local read "PWMTaskA"() -> (w164:refnum<k21>)
        n146 = local read "PWMTaskC"() -> (w137:refnum<k21>)
        n147 = local read "PWMTaskB"() -> (w162:refnum<k21>)
        n148 = local read "LoopFreq(Hz)"() -> (w118:dbl)
        n149 = expression code="(1/x)*1e6"(w118) -> (w117:dbl)
        n150 = call-poly <vilib>:"DAQmx Write.vi"("task/channels in"=w164, "frequency"=w115, "duty cycle"=w153) -> ()  [unwired: 10 in, 3 out]
        n151 = call-poly <vilib>:"DAQmx Write.vi"("task/channels in"=w162, "frequency"=w115, "duty cycle"=w152) -> ()  [unwired: 10 in, 3 out]
        n152 = call-poly <vilib>:"DAQmx Write.vi"("task/channels in"=w137, "frequency"=w115, "duty cycle"=w151) -> ()  [unwired: 10 in, 3 out]
        n153 = local read "stop"() -> (w148:bool)
        n154 = node-c288(w117) -> ()  [unwired: 1 out]
      }
      n155 = node-c288(w82) -> ()  [unwired: 1 out]
    }
    frame #3 {
      n156 = local read "PWMTaskA"() -> (w212:refnum<k21>)
      n157 = local read "PWMTaskC"() -> (w204:refnum<k21>)
      n158 = local read "PWMTaskB"() -> (w210:refnum<k21>)
      n159 = call <vilib>:"DAQmx Stop Task.vi"("task/channels in"=refnum<k21> "ForceInABC") -> ("error out"=w215:errorcluster)  [unwired: 13 in, 1 out]
      n160 = call <vilib>:"DAQmx Stop Task.vi"("task/channels in"=refnum<k21> "MotorDirABC") -> ("error out"=w216:errorcluster)  [unwired: 13 in, 1 out]
      n161 = call <vilib>:"DAQmx Clear Task.vi"("task in"=w212) -> ("error out"=w217:errorcluster)  [unwired: 14 in]
      n162 = call <vilib>:"DAQmx Clear Task.vi"("task in"=w210) -> ("error out"=w209:errorcluster)  [unwired: 14 in]
      n163 = call <vilib>:"DAQmx Clear Task.vi"("task in"=w204) -> ("error out"=w205:errorcluster)  [unwired: 14 in]
      n164 = call <vilib>:"DAQmx Stop Task.vi"("task/channels in"=refnum<k21> "PositionInA") -> ("error out"=w218:errorcluster)  [unwired: 13 in, 1 out]
      n165 = call <vilib>:"DAQmx Stop Task.vi"("task/channels in"=refnum<k21> "PositionInB") -> ("error out"=w207:errorcluster)  [unwired: 13 in, 1 out]
      n166 = call <vilib>:"DAQmx Stop Task.vi"("task/channels in"=refnum<k21> "PositionInC") -> ("error out"=w203:errorcluster)  [unwired: 13 in, 1 out]
      n167 = local write "stop"(FALSE ("stop")) -> ()
      n168 = call <vilib>:"General Error Handler.vi"("error in (no error)"=w215) -> ()  [unwired: 10 in, 5 out]
      n169 = call <vilib>:"General Error Handler.vi"("error in (no error)"=w216) -> ()  [unwired: 10 in, 5 out]
      n170 = call <vilib>:"General Error Handler.vi"("error in (no error)"=w217) -> ()  [unwired: 10 in, 5 out]
      n171 = call <vilib>:"General Error Handler.vi"("error in (no error)"=w209) -> ()  [unwired: 10 in, 5 out]
      n172 = call <vilib>:"General Error Handler.vi"("error in (no error)"=w205) -> ()  [unwired: 10 in, 5 out]
      n173 = call <vilib>:"General Error Handler.vi"("error in (no error)"=w218) -> ()  [unwired: 10 in, 5 out]
      n174 = call <vilib>:"General Error Handler.vi"("error in (no error)"=w207) -> ()  [unwired: 10 in, 5 out]
      n175 = call <vilib>:"General Error Handler.vi"("error in (no error)"=w203) -> ()  [unwired: 10 in, 5 out]
    }
  }
